vi "HW_GEN - Genrate Active Module Configurations.vi"(8 "错误输入":errorcluster caption="错误输入（无错误）", 9 "ModInfo in":T1, 10 "HWdef":path, 11 "HWcfg Path":path) -> (0 "错误输出":errorcluster, 2 "Chan dflt Para out":T6, 3 "ModuCfg":T3)   [LabVIEW 2016]
uses:
  ToolKit/Popup/Private/Ctrls/POP_Data Type.ctl
  Ctrls/HardWare _ Channel Configurations PopUp Type.ctl
  Ctrls/HardWare _ Module Configuration.ctl
  Ctrls/HardWare Basic Info _ Channel.ctl
  Ctrls/HardWare Basic Info _ Module.ctl
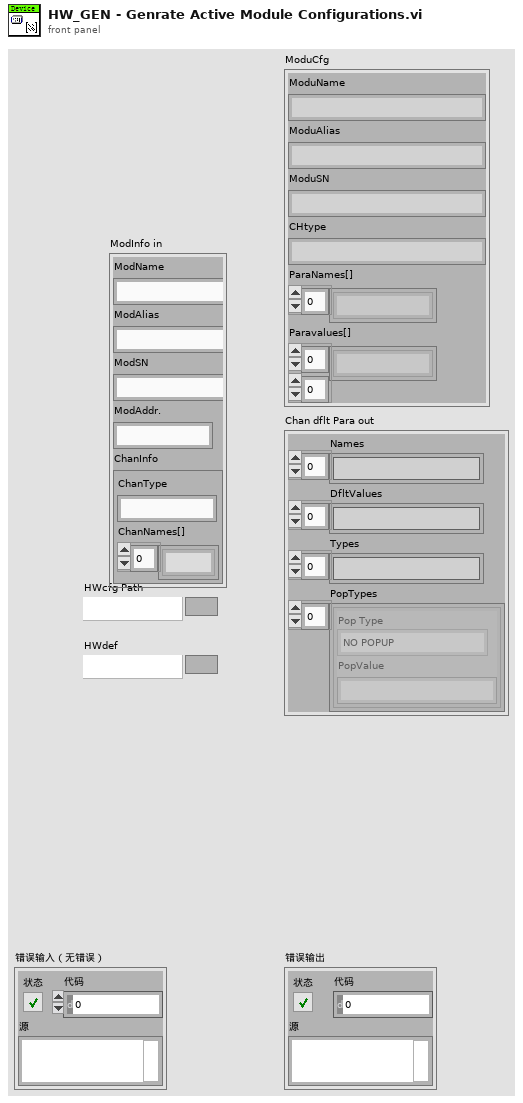
[diagram p1: front panel]
types:
  T1 = typedef "HardWare Basic Info _ Module.ctl" = cluster{"ModName":string, "ModAlias":string, "ModSN":string, "ModAddr.":string, "ChanInfo":T2}
  T2 = typedef "HardWare Basic Info _ Channel.ctl" = cluster{"ChanType":string, "ChanNames[]":string[]}
  T3 = typedef "HardWare _ Module Configuration.ctl" = cluster{"ModuName":string, "ModuAlias":string, "ModuSN":string, "CHtype":string, "ParaNames[]":string[], "Paravalues[]":string[][]}
  T4 = typedef "HardWare _ Channel Configurations PopUp Type.ctl" = cluster{"Pop Type":T5, "PopValue":string}
  T5 = typedef "POP_Data Type.ctl" = enum16{"NO POPUP", "Unkown", "String", "Integer", "Float", "Color", "Boolean", "Ring", "Captioned String", "Captioned Integer", "Button Color", "2 Int Cluster", "4 Int Cluster", "6-Dbl Cluster", "Path", "Combox", "Time", "ShotCut String"}
  T6 = cluster{"Names":string[], "DfltValues":string[], "Types":string[], "PopTypes":T4[]}
  T7 = cluster{"ParaNames":string[], "DfltPara":string[], "Types":string[], "PopTypes":T4[]}
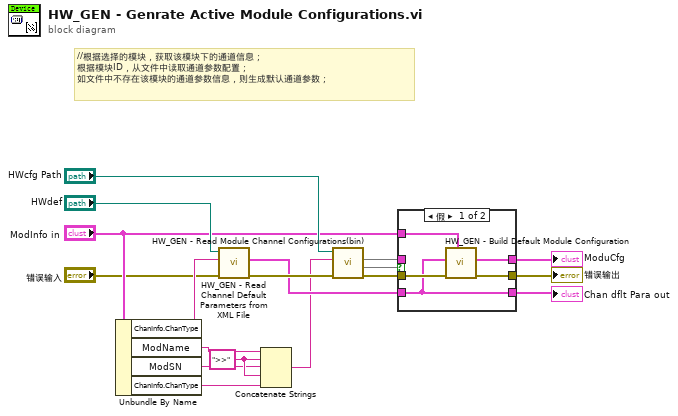
[diagram p0: block diagram]
diagram:
  w5 = ">>" ("string")
  # "//根据选择的模块，获取该模块下的通道信息；\n根据模块ID，从文件中读取通道参数配置；\n如文件中不存在该模块的通道参数信息，则生成默认通道参数；"
  n1 = Unbundle By Name("ModInfo in") -> ("ChanInfo.ChanType"=w9:string, "ModName"=w4:string, "ModSN"=w3:string, "ChanInfo.ChanType"=w2:string)
  n2 = call "HW_GEN - Read Channel Default Parameters from XML File.vi"("error in"="错误输入", "ChanType"=w9, "path to XML document"="HWdef") -> ("错误输出"=w15:errorcluster, "Chan dflt Para out"=w13:T7)  [unwired: 7 in]
  n3 = Concatenate Strings(w4, w5, w3, w5, w2) -> (w1:string)
  n4 = call "HW_GEN - Read Module Channel Configurations(bin).vi"("error in"=w15, 10:w1, "ModuCFG path"="HWcfg Path") -> ("error out"=w16:errorcluster, 1:w10, 2:w14)  [unwired: 5 in, 1 out]
  n5 = case shown="假" w10 {
    tunnel: w14 -> [_ w26]
    tunnel: [w23 w26] -> w11
    tunnel: w13 -> [w19 w24]
    tunnel: w16 -> [w20 w25]
    tunnel: [w22 w25] -> w12
    tunnel: "ModInfo in" -> [w21 _]
    tunnel: [w19 w24] -> w18
    frame False {
      n6 = call "HW_GEN - Build Default Module Configuration.vi"("ModInfo"=w21, "error in"=w20, "Chan dflt Para in"=w19) -> ("error out"=w22:errorcluster, "ModuCfg"=w23:T3)  [unwired: 7 in]
    }
    frame True {
    }
  }
  "Chan dflt Para out" <- w18
  "错误输出" <- w12
  "ModuCfg" <- w11
